vi "FilterNodesByRef.vi"(8 "error in":errorcluster, 10 "NISE_CEF_Node":refnum<class "NISE_CEF_Node.lvclass">, 11 "nodes":refnum<data-value>[](array[refnum])) -> (0 "error out":errorcluster, 3 "filtered nodes":refnum<data-value>[](array[refnum]))   [LabVIEW 2013, in "NISE_CEF_Node.lvclass"]
uses:
  NISE_CEF_Node.lvclass
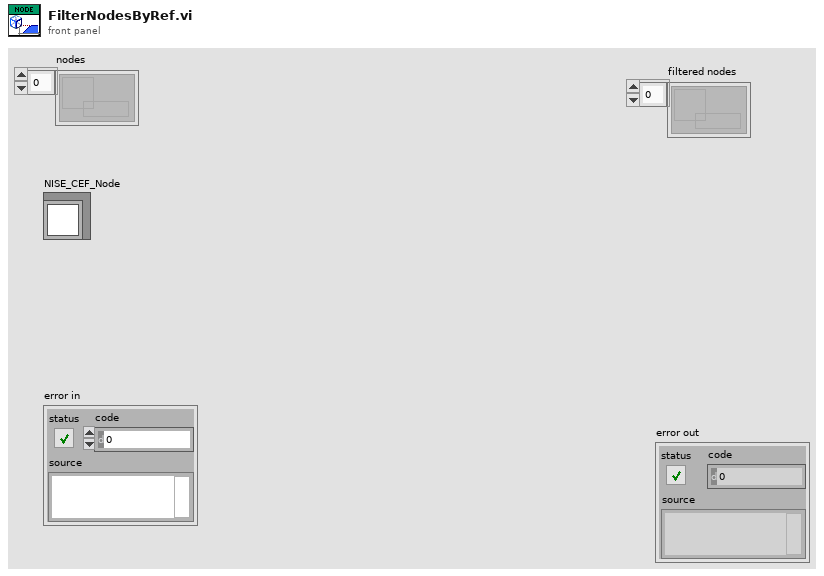
[diagram p1: front panel]
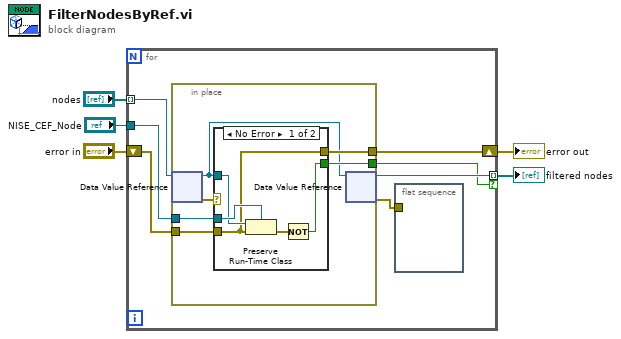
[diagram p0: block diagram]
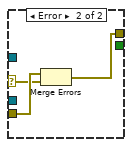
[diagram p2: hidden frame]
diagram:
  n1 = for {
    shift-right: [w11] -> w4
    shift-left: "error in" -> [w12]
    tunnel: "nodes" -> [w9] mode=indexing
    tunnel: [w8] -> w2 mode=indexing if=w6
    tunnel: "NISE_CEF_Node" -> [w10]
    n2 = in-place {
      in-place-border: w12 -> [w18]
      in-place-border: [w17] -> w11
      in-place-border: w10 -> [w16]
      in-place-border: [w14] -> w6
      n3 = in-place-dvr #1(w9) -> (w13:refnum<class "NISE_CEF_Node.lvclass">, w15:errorcluster)
      n4 = case shown="No Error" w15 {
        selector: w15 -> [_ w24]
        tunnel: w18 -> [w21 w26]
        tunnel: [w21 w25] -> w17
        tunnel: w16 -> [w23 _]
        tunnel: w13 -> [w22 _]
        tunnel: [w19 _] -> w14
        frame No Error {
          n5 = Preserve Run-Time Class(object in=w22, error in=w21, 2:w23) -> (error out=w20:errorcluster)  [unwired: 1 out]
          n6 = Not(x=w20) -> (.not. x?=w19:bool)
        }
        frame Error {
          n7 = Merge Errors(w26, w24) -> (w25:errorcluster)
        }
      }
      n8 = in-place-dvr #1(w13) -> (w8:refnum<data-value>, w7:errorcluster)
    }
    n9 = flat-sequence {
      tunnel: w7 -> [_]
      frame #0 {
      }
    }
  }
  "error out" <- w4
  "filtered nodes" <- w2
